vi "Encoder_PWM.vi"() -> ()   [LabVIEW 2019]
uses:
  <vilib>/rvi/Emulation/niFpgaGetClockAttributes.vi
  <vilib>/rvi/Emulation/niFpgaSctlEmulationGetInTimedLoop.vi
  <vilib>/rvi/Emulation/niFpgaEmulationReportErrorSimple.vi
  <vilib>/rvi/Emulation/niFpgaProcessEmulError.vi
  <vilib>/rvi/eio/common/nirviEmuTemplateMethod_errors.vi
  <vilib>/rvi/Emulation/niFpgaCriticalErrorInLSC.vi
  <vilib>/eio/EIONode/EIONode.xnode
panel:
  in  "ena 3":bool
  in  "ena 2":bool
  in  "실린더 후진":bool
  in  "실린더 전진":bool
  out "오른쪽Y 아래":bool
  out "오른쪽Y 위":bool
  out "오른쪽X 오른쪽":bool
  out "오른쪽X 왼쪽":bool
  out "왼쪽Y아래":bool
  out "왼쪽Y위":bool
  out "왼쪽x오른쪽":bool
  out "왼쪽x왼쪽":bool
  in  "오른쪽 바퀴 입력":i16
  out "Enc 3":i32
  in  "Enc_Reset 3":bool
  in  "Homing Value 3":i32
  in  "?":bool
  out "Enc 2":i32
  in  "Enc_Reset 2":bool
  in  "Homing Value 2":i32
  in  "?":bool
  in  "왼쪽 바퀴 입력":i16
  out "비상정지":bool
  in  "?":bool
  in  "ena":bool
  in  "PWM 90%":i16=18000
  in  "PWM 10%":i16=2000
  in  "PWM Freq":i16=20000
  in  "도르래 입력":i16
  out "Enc":i32
  in  "Enc_Reset":bool
  in  "Homing Value":i32
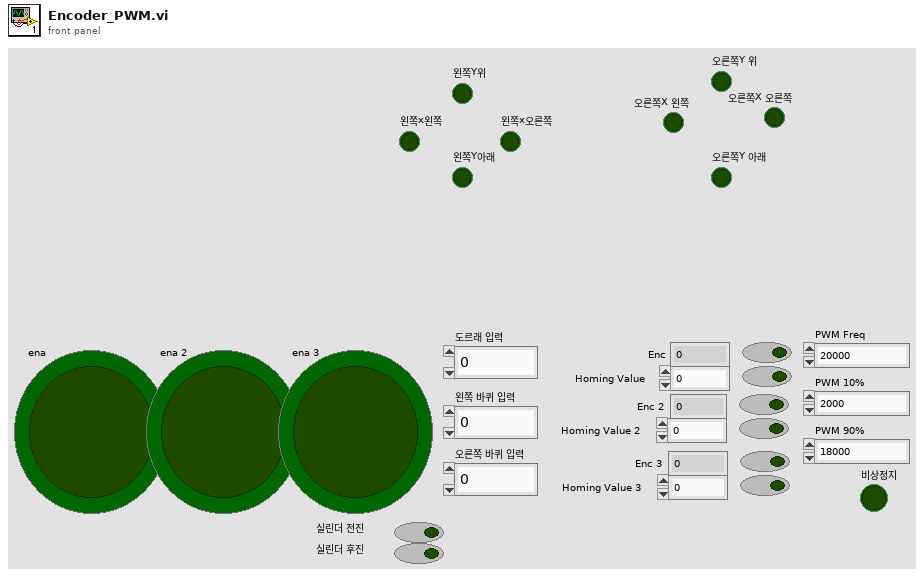
[diagram p1: front panel]
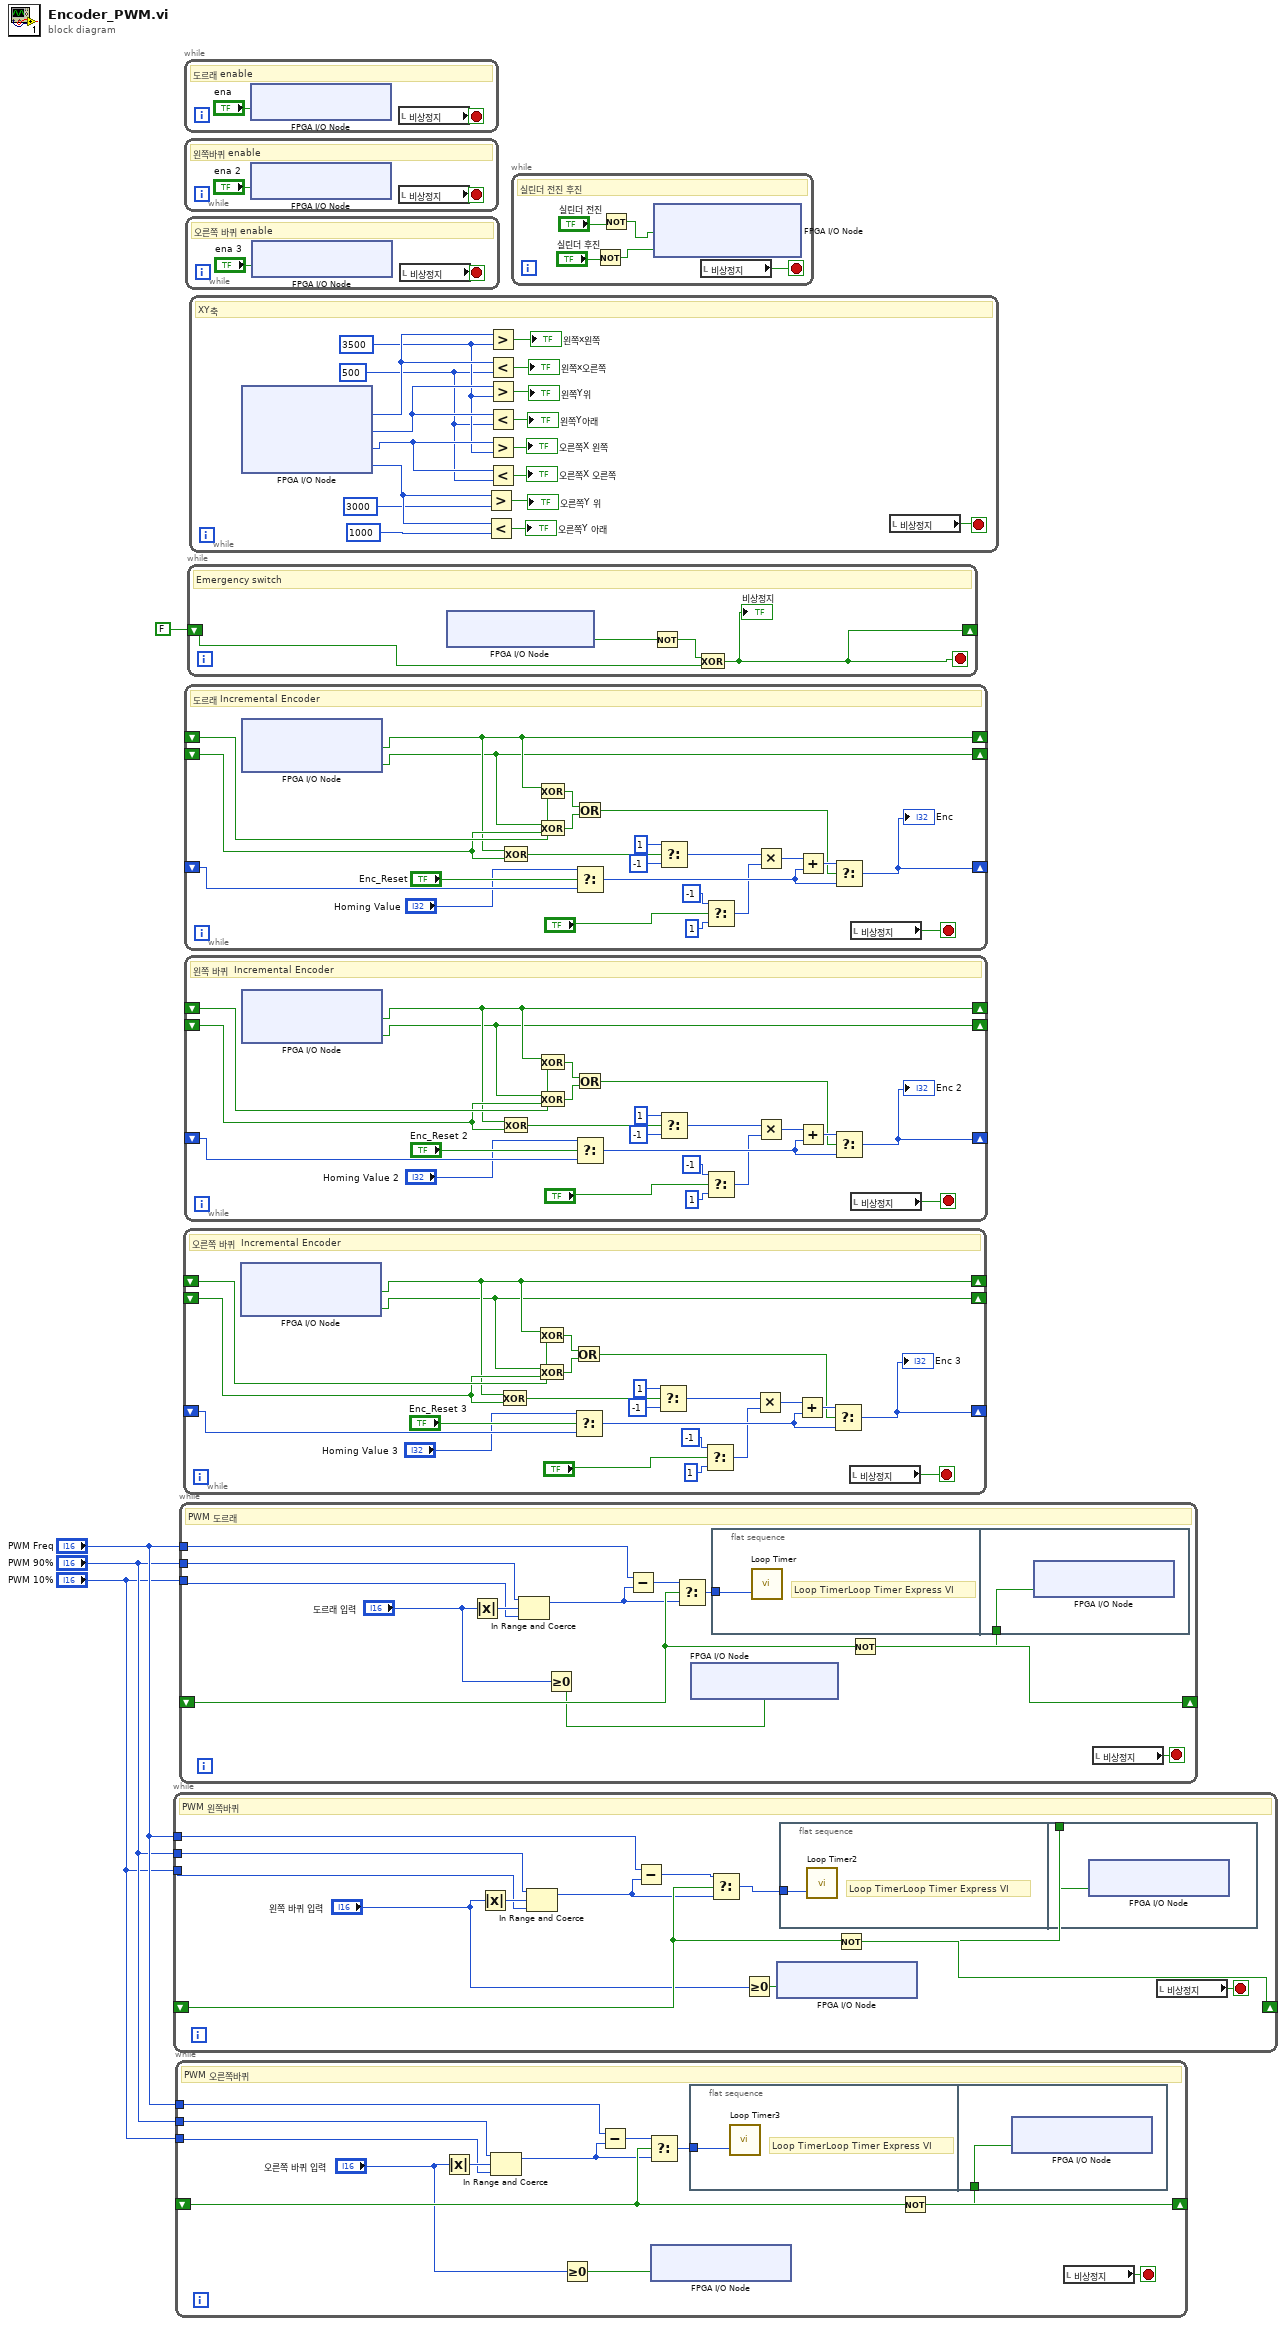
[diagram p0: block diagram]
diagram:
  n1 = while "PWM Generation" {
    shift-right: [w15] -> _
    shift-left: _ -> [w13]
    tunnel: "PWM 10%" -> [w10]
    tunnel: "PWM Freq" -> [w12]
    tunnel: "PWM 90%" -> [w9]
    stop <- w7 stop-if-true
    # "PWM 왼쪽바퀴"
    n2 = Absolute Value(x="왼쪽 바퀴 입력") -> (abs(x)=w11:i16)
    n3 = In Range and Coerce(upper limit=w9, x=w11, lower limit=w10) -> (coerced(x)=w8:i16)  [unwired: 1 out]
    n4 = Subtract(x=w12, y=w8) -> (x-y=w14:i16)
    n5 = Select(t=w14, s=w13, f=w8) -> (s? t:f=w16:i16)
    n6 = Greater Or Equal To 0?(x="왼쪽 바퀴 입력") -> (x >= 0?=w6:bool)
    n7 = xnode "FPGA I/O Node"("ConnectorC/DIO0"=w6) -> ()  [unwired: 1 in, 1 out]
    n8 = flat-sequence {
      tunnel: w16 -> [w17]
      tunnel: w13 -> [w18]
      frame #0 {
        # "Loop TimerLoop Timer Express VI"
        n9 = call "Loop Timer2"("Count(Ticks)"=w17) -> ()  [unwired: 1 out]
      }
      frame #1 {
        n10 = xnode "FPGA I/O Node"("ConnectorA/DIO7"=w18) -> ()  [unwired: 1 in, 1 out]
      }
    }
    n11 = Not(x=w13) -> (.not. x?=w15:bool)
    n12 = local read "비상정지"() -> (w7:bool)
  }
  n13 = while "PWM Generation" {
    shift-right: [w29] -> _
    shift-left: _ -> [w27]
    tunnel: "PWM 10%" -> [w24]
    tunnel: "PWM Freq" -> [w26]
    tunnel: "PWM 90%" -> [w23]
    stop <- w21 stop-if-true
    # "PWM 오른쪽바퀴"
    n14 = Absolute Value(x="오른쪽 바퀴 입력") -> (abs(x)=w25:i16)
    n15 = In Range and Coerce(upper limit=w23, x=w25, lower limit=w24) -> (coerced(x)=w22:i16)  [unwired: 1 out]
    n16 = Greater Or Equal To 0?(x="오른쪽 바퀴 입력") -> (x >= 0?=w20:bool)
    n17 = Subtract(x=w26, y=w22) -> (x-y=w28:i16)
    n18 = Select(t=w28, s=w27, f=w22) -> (s? t:f=w30:i16)
    n19 = xnode "FPGA I/O Node"("ConnectorC/DIO1"=w20) -> ()  [unwired: 1 in, 1 out]
    n20 = flat-sequence {
      tunnel: w30 -> [w31]
      tunnel: w27 -> [w32]
      frame #0 {
        # "Loop TimerLoop Timer Express VI"
        n21 = call "Loop Timer3"("Count(Ticks)"=w31) -> ()  [unwired: 1 out]
      }
      frame #1 {
        n22 = xnode "FPGA I/O Node"("ConnectorA/DIO8"=w32) -> ()  [unwired: 1 in, 1 out]
      }
    }
    n23 = Not(x=w27) -> (.not. x?=w29:bool)
    n24 = local read "비상정지"() -> (w21:bool)
  }
  n25 = while "PWM Generation" {
    shift-right: [w43] -> _
    shift-left: _ -> [w41]
    tunnel: "PWM 10%" -> [w38]
    tunnel: "PWM Freq" -> [w40]
    tunnel: "PWM 90%" -> [w37]
    stop <- w35 stop-if-true
    # "PWM 도르래"
    n26 = Absolute Value(x="도르래 입력") -> (abs(x)=w39:i16)
    n27 = In Range and Coerce(upper limit=w37, x=w39, lower limit=w38) -> (coerced(x)=w36:i16)  [unwired: 1 out]
    n28 = Greater Or Equal To 0?(x="도르래 입력") -> (x >= 0?=w34:bool)
    n29 = Subtract(x=w40, y=w36) -> (x-y=w42:i16)
    n30 = Select(t=w42, s=w41, f=w36) -> (s? t:f=w44:i16)
    n31 = xnode "FPGA I/O Node"("ConnectorA/DIO14"=w34) -> ()  [unwired: 1 in, 1 out]
    n32 = flat-sequence {
      tunnel: w44 -> [w45]
      tunnel: w41 -> [w46]
      frame #0 {
        # "Loop TimerLoop Timer Express VI"
        n33 = call "Loop Timer"("Count(Ticks)"=w45) -> ()  [unwired: 1 out]
      }
      frame #1 {
        n34 = xnode "FPGA I/O Node"("ConnectorA/DIO6"=w46) -> ()  [unwired: 1 in, 1 out]
      }
    }
    n35 = Not(x=w41) -> (.not. x?=w43:bool)
    n36 = local read "비상정지"() -> (w35:bool)
  }
  n37 = while {
    shift-right: [w50] -> _
    shift-left: _ -> [w58]
    shift-right: [w49] -> _
    shift-left: _ -> [w57]
    shift-right: [w60] -> _
    shift-left: _ -> [w59]
    stop <- w47 stop-if-true
    # "오른쪽 바퀴  Incremental Encoder"
    n38 = xnode "FPGA I/O Node"() -> ("ConnectorA/DIO4"=w50:bool, "ConnectorA/DIO5"=w49:bool)  [unwired: 2 in, 2 out]
    n39 = Exclusive Or(1:w57, 2:w50) -> (0:w62:bool)
    n40 = Exclusive Or(1:w58, 2:w50) -> (0:w64:bool)
    n41 = Exclusive Or(1:w57, 2:w49) -> (0:w65:bool)
    n42 = Or(x=w64, y=w65) -> (x .or. y?=w63:bool)
    n43 = Select(t="Homing Value 3", s="Enc_Reset 3", f=w59) -> (s? t:f=w68:i32)
    n44 = Select(t=i8 1 ("16 bit"), s=w62, f=i8 -1 ("16 bit")) -> (s? t:f=w53:i8)
    n45 = Select(t=i8 -1 ("16 bit"), s="?", f=i8 1 ("16 bit")) -> (s? t:f=w52:i8)
    n46 = Multiply(x=w53, y=w52) -> (x*y=w51:i8)
    n47 = Add(x=w51, y=w68) -> (x+y=w69:i32)
    n48 = Select(t=w69, s=w63, f=w68) -> (s? t:f=w60:i32)
    "Enc 3" <- w60
    n49 = local read "비상정지"() -> (w47:bool)
  }
  n50 = while {
    stop <- w71 stop-if-true
    # "도르래 enable"
    n51 = xnode "FPGA I/O Node"("ConnectorC/DIO2"="ena") -> ()  [unwired: 1 in, 1 out]
    n52 = local read "비상정지"() -> (w71:bool)
  }
  n53 = while {
    stop <- w73 stop-if-true
    # "왼쪽바퀴 enable"
    n54 = xnode "FPGA I/O Node"("ConnectorC/DIO3"="ena 2") -> ()  [unwired: 1 in, 1 out]
    n55 = local read "비상정지"() -> (w73:bool)
  }
  n56 = while {
    shift-right: [w77] -> _
    shift-left: _ -> [w85]
    shift-right: [w76] -> _
    shift-left: _ -> [w84]
    shift-right: [w87] -> _
    shift-left: _ -> [w86]
    stop <- w74 stop-if-true
    # "도르래 Incremental Encoder"
    n57 = xnode "FPGA I/O Node"() -> ("ConnectorA/DIO0"=w77:bool, "ConnectorA/DIO1"=w76:bool)  [unwired: 2 in, 2 out]
    n58 = Exclusive Or(1:w84, 2:w77) -> (0:w89:bool)
    n59 = Exclusive Or(1:w85, 2:w77) -> (0:w91:bool)
    n60 = Exclusive Or(1:w84, 2:w76) -> (0:w92:bool)
    n61 = Or(x=w91, y=w92) -> (x .or. y?=w90:bool)
    n62 = Select(t="Homing Value", s="Enc_Reset", f=w86) -> (s? t:f=w95:i32)
    n63 = Select(t=i8 1 ("16 bit"), s=w89, f=i8 -1 ("16 bit")) -> (s? t:f=w80:i8)
    n64 = Select(t=i8 -1 ("16 bit"), s="?", f=i8 1 ("16 bit")) -> (s? t:f=w79:i8)
    n65 = Multiply(x=w80, y=w79) -> (x*y=w78:i8)
    n66 = Add(x=w78, y=w95) -> (x+y=w96:i32)
    n67 = Select(t=w96, s=w90, f=w95) -> (s? t:f=w87:i32)
    "Enc" <- w87
    n68 = local read "비상정지"() -> (w74:bool)
  }
  n69 = while {
    shift-right: [w100] -> _
    shift-left: _ -> [w108]
    shift-right: [w99] -> _
    shift-left: _ -> [w107]
    shift-right: [w110] -> _
    shift-left: _ -> [w109]
    stop <- w97 stop-if-true
    # "왼쪽 바퀴  Incremental Encoder"
    n70 = xnode "FPGA I/O Node"() -> ("ConnectorA/DIO2"=w100:bool, "ConnectorA/DIO3"=w99:bool)  [unwired: 2 in, 2 out]
    n71 = Exclusive Or(1:w107, 2:w100) -> (0:w112:bool)
    n72 = Exclusive Or(1:w108, 2:w100) -> (0:w114:bool)
    n73 = Exclusive Or(1:w107, 2:w99) -> (0:w115:bool)
    n74 = Or(x=w114, y=w115) -> (x .or. y?=w113:bool)
    n75 = Select(t="Homing Value 2", s="Enc_Reset 2", f=w109) -> (s? t:f=w118:i32)
    n76 = Select(t=i8 1 ("16 bit"), s=w112, f=i8 -1 ("16 bit")) -> (s? t:f=w103:i8)
    n77 = Select(t=i8 -1 ("16 bit"), s="?", f=i8 1 ("16 bit")) -> (s? t:f=w102:i8)
    n78 = Multiply(x=w103, y=w102) -> (x*y=w101:i8)
    n79 = Add(x=w101, y=w118) -> (x+y=w119:i32)
    n80 = Select(t=w119, s=w113, f=w118) -> (s? t:f=w110:i32)
    "Enc 2" <- w110
    n81 = local read "비상정지"() -> (w97:bool)
  }
  n82 = while {
    stop <- w121 stop-if-true
    # "오른쪽 바퀴 enable"
    n83 = xnode "FPGA I/O Node"("ConnectorC/DIO4"="ena 3") -> ()  [unwired: 1 in, 1 out]
    n84 = local read "비상정지"() -> (w121:bool)
  }
  n85 = while {
    shift-right: [w122] -> _
    shift-left: FALSE -> [w124]
    stop <- w122 stop-if-true
    # "Emergency switch"
    n86 = xnode "FPGA I/O Node"() -> ("ConnectorA/DIO13"=w125:bool)  [unwired: 1 in, 1 out]
    n87 = Not(x=w125) -> (.not. x?=w123:bool)
    n88 = Exclusive Or(1:w124, 2:w123) -> (0:w122:bool)
    "비상정지" <- w122
  }
  n89 = while {
    stop <- w130 stop-if-true
    w127 = i16 3500
    w126 = i16 500
    # "XY축"
    n90 = xnode "FPGA I/O Node"() -> ("ConnectorA/AI0"=w134:u16, "ConnectorA/AI1"=w133:u16, "ConnectorA/AI2"=w132:u16, "ConnectorA/AI3"=w131:u16)  [unwired: 4 in, 4 out]
    n91 = Greater?(x=w131, y=i16 3000) -> (0:→"오른쪽Y 위":bool)
    n92 = Less?(x=w131, y=i16 1000) -> (x < y?=→"오른쪽Y 아래":bool)
    n93 = Greater?(x=w134, y=w127) -> (0:→"왼쪽x왼쪽":bool)
    n94 = Less?(x=w134, y=w126) -> (x < y?=→"왼쪽x오른쪽":bool)
    n95 = Greater?(x=w133, y=w127) -> (0:→"왼쪽Y위":bool)
    n96 = Less?(x=w133, y=w126) -> (x < y?=→"왼쪽Y아래":bool)
    n97 = Greater?(x=w132, y=w127) -> (0:→"오른쪽X 왼쪽":bool)
    n98 = Less?(x=w132, y=w126) -> (x < y?=→"오른쪽X 오른쪽":bool)
    n99 = local read "비상정지"() -> (w130:bool)
  }
  n100 = while {
    stop <- w143 stop-if-true
    # "실린더 전진 후진"
    n101 = Not(x="실린더 후진") -> (.not. x?=w146:bool)
    n102 = Not(x="실린더 전진") -> (.not. x?=w145:bool)
    n103 = xnode "FPGA I/O Node"("ConnectorA/DIO11"=w145, "ConnectorA/DIO15"=w146) -> ()  [unwired: 2 in, 2 out]
    n104 = local read "비상정지"() -> (w143:bool)
  }
